vi "IB_RW_Project_Destinations.vi"(7 "action":T2, 8 "ErrIn":errorcluster, 9 "index":string, 10 "data":T1, 11 "buildObject":T3) -> (0 "ErrOut":errorcluster, 1 "index out":string, 2 "data":T1, 3 "buildObject out":T3)   [LabVIEW 2020]
uses:
  <resource>/Framework/Providers/API/ItemRef.ctl
  <vilib>/AppBuilder/IB_RW_Project/IB_RW_Project_PropBag_Action.ctl
  <vilib>/AppBuilder/IB_RW_Project/IB_RW_Project_Destination_Data.ctl
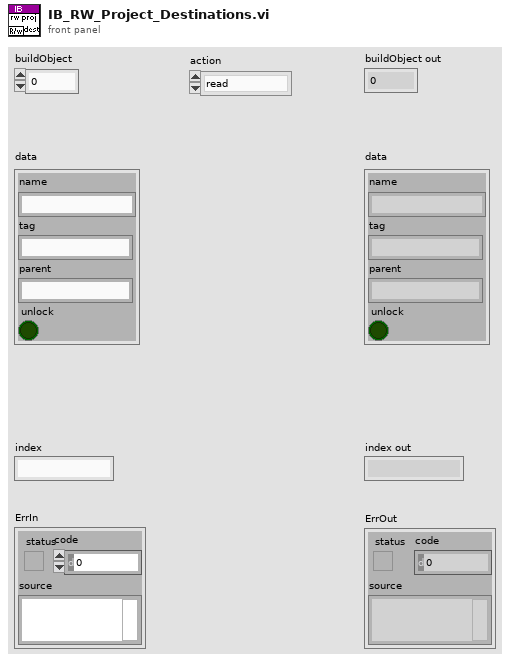
[diagram p1: front panel]
types:
  T1 = typedef "IB_RW_Project_Destination_Data.ctl" = cluster{"name":string, "tag":string, "parent":string, "unlock":bool}
  T2 = typedef "IB_RW_Project_PropBag_Action.ctl" = enum16{"read", "write", "clear", "readPrevious", "writePrevious", "clearPrevious"}
  T3 = typedef "ItemRef.ctl" = u64
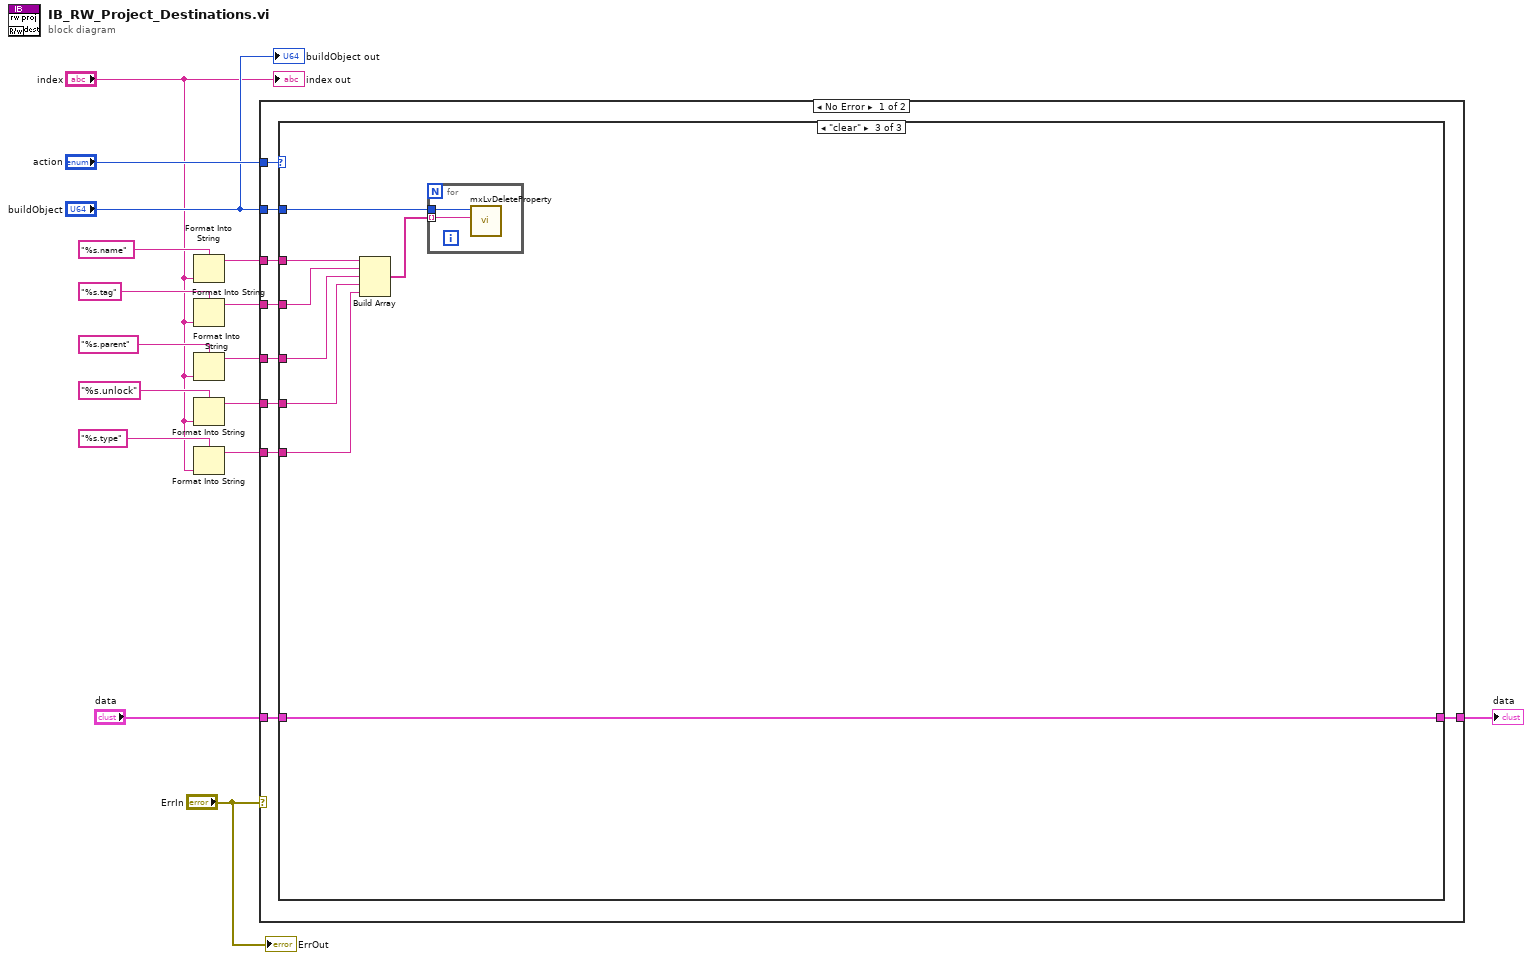
[diagram p0: block diagram]
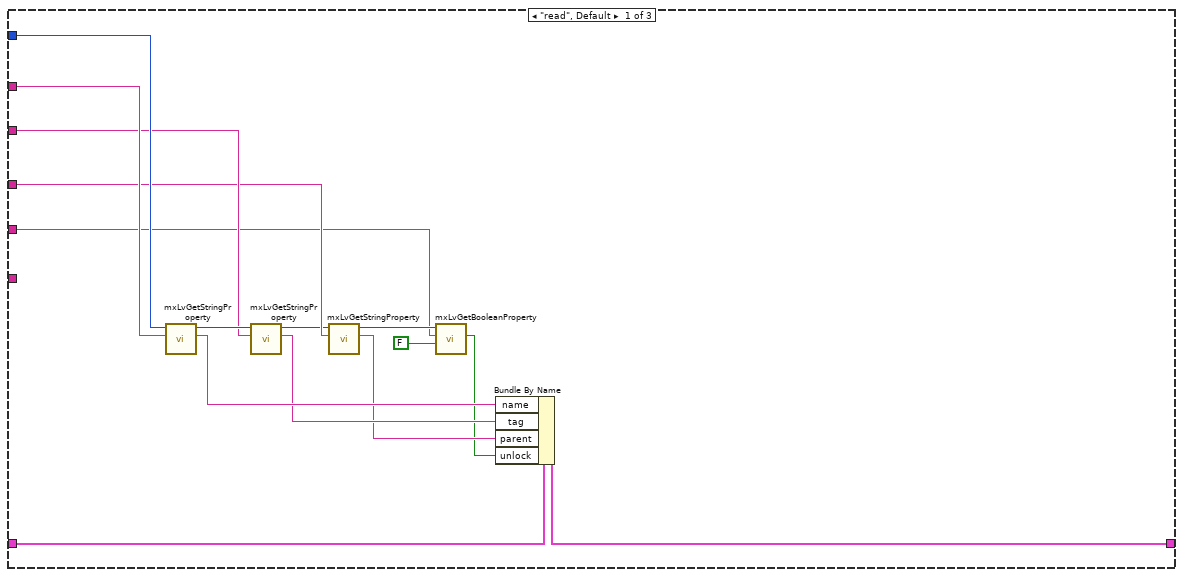
[diagram p2: hidden frame]
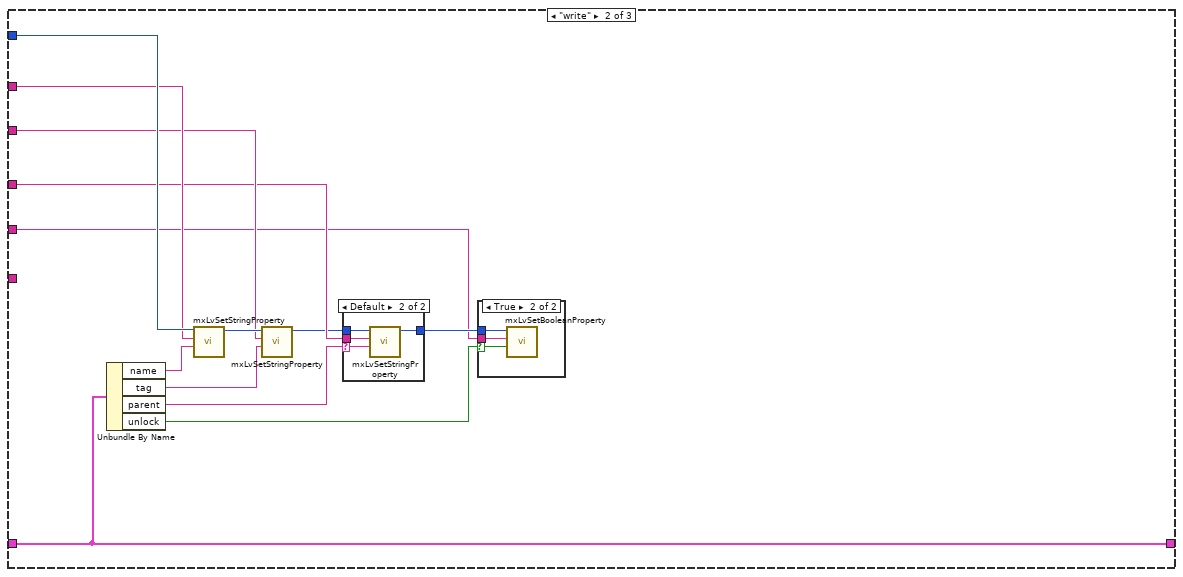
[diagram p3: hidden frame]
diagram:
  n1 = Format Into String(format string="%s.name", "index") -> (resulting string=w11:string)  [unwired: 2 in, 1 out]
  n2 = Format Into String(format string="%s.tag", "index") -> (resulting string=w10:string)  [unwired: 2 in, 1 out]
  n3 = Format Into String(format string="%s.parent", "index") -> (resulting string=w8:string)  [unwired: 2 in, 1 out]
  n4 = Format Into String(format string="%s.unlock", "index") -> (resulting string=w5:string)  [unwired: 2 in, 1 out]
  n5 = Format Into String(format string="%s.type", "index") -> (resulting string=w1:string)  [unwired: 2 in, 1 out]
  n6 = case shown="No Error" "ErrIn" {
    tunnel: "action" -> [w25 _]
    tunnel: "buildObject" -> [w24 _]
    tunnel: "data" -> [w23 w72]
    tunnel: [w22 w72] -> w7
    tunnel: w11 -> [w21 _]
    tunnel: w10 -> [w20 _]
    tunnel: w8 -> [w19 _]
    tunnel: w5 -> [w18 _]
    tunnel: w1 -> [w17 _]
    frame No Error {
      n7 = case shown="\"clear\"" w25 {
        tunnel: w24 -> [w38 w49 w69]
        tunnel: w23 -> [w32 w50 w63]
        tunnel: [w31 w50 w63] -> w22
        tunnel: w21 -> [w37 w48 w68]
        tunnel: w20 -> [w35 w47 w67]
        tunnel: w19 -> [w34 w45 w66]
        tunnel: w18 -> [w33 w43 w64]
        tunnel: w17 -> [_ _ w62]
        frame "read", Default {
          n8 = call <resource>:"mxLvGetStringProperty.vi"("Tag"=w37, "Item"=w38) -> ("Value"=w30:string, "Item"=w40:T3)  [unwired: 1 in, 7 out]
          n9 = call <resource>:"mxLvGetStringProperty.vi"("Tag"=w35, "Item"=w40) -> ("Value"=w29:string, "Item"=w26:T3)  [unwired: 1 in, 7 out]
          n10 = call <resource>:"mxLvGetStringProperty.vi"("Tag"=w34, "Item"=w26) -> ("Value"=w28:string, "Item"=w36:T3)  [unwired: 1 in, 7 out]
          n11 = call <resource>:"mxLvGetBooleanProperty.vi"("Default Value (F)"=FALSE, "Tag"=w33, "Item"=w36) -> ("Value"=w27:bool)  [unwired: 1 in, 7 out]
          n12 = Bundle By Name(cluster=w32, "name"=w30, "tag"=w29, "parent"=w28, "unlock"=w27) -> (w31:T1)
        }
        frame "write" {
          n13 = Unbundle By Name(w50) -> ("name"=w51:string, "tag"=w52:string, "parent"=w41:string, "unlock"=w44:bool)
          n14 = call <resource>:"mxLvSetStringProperty.vi"("Value (\"\")"=w51, "Tag"=w48, "Item"=w49) -> ("Item"=w53:T3)  [unwired: 2 in, 6 out]
          n15 = call <resource>:"mxLvSetStringProperty.vi"("Value (\"\")"=w52, "Tag"=w47, "Item"=w53) -> ("Item"=w42:T3)  [unwired: 2 in, 6 out]
          n16 = case shown="Default" w41 {
            selector: w41 -> [_ w55]
            tunnel: [w54 w58] -> w46
            tunnel: w45 -> [_ w57]
            tunnel: w42 -> [w54 w56]
            frame "" {
            }
            frame Default {
              n17 = call <resource>:"mxLvSetStringProperty.vi"("Value (\"\")"=w55, "Tag"=w57, "Item"=w56) -> ("Item"=w58:T3)  [unwired: 2 in, 6 out]
            }
          }
          n18 = case shown="True" w44 {
            selector: w44 -> [_ w59]
            tunnel: w46 -> [_ w61]
            tunnel: w43 -> [_ w60]
            frame False {
            }
            frame True {
              n19 = call <resource>:"mxLvSetBooleanProperty.vi"("Value (F)"=w59, "Tag"=w60, "Item"=w61) -> ()  [unwired: 2 in, 7 out]
            }
          }
        }
        frame "clear" {
          n20 = Build Array(w68, w67, w66, w64, w62) -> (w65:string[])
          n21 = for {
            tunnel: w69 -> [w71]
            tunnel: w65 -> [w70] mode=indexing
            n22 = call <resource>:"mxLvDeleteProperty.vi"("Tag"=w70, "Item"=w71) -> ()  [unwired: 1 in, 9 out]
          }
        }
      }
    }
    frame Error {
    }
  }
  "data" <- w7
  "buildObject out" <- "buildObject"
  "ErrOut" <- "ErrIn"
  "index out" <- "index"
